vi "GCSArray_regex_select.vi"(0 "GCSArray input string":string, 1 "Selector":T2, 2 "Range":T1, 5 "error in (no error)":errorcluster) -> (14 "Matches":T1[](array[typedef]), 19 "error out":errorcluster)   [LabVIEW 2026]
doc: "Performs the same task as GCSArray_regex_matches.vi, but it returns the found indices as an array of range objects instead of an array of text strings."
uses:
  GCSArray_regex_selector.ctl
  GCSArray_regex_range.ctl
  <vilib>/regexp/Match Regular Expression.xnode
panel:
  # "Select parts ('Selector') of a GCSArray ('Input string')\nand return all found entry ranges ('Matches')."
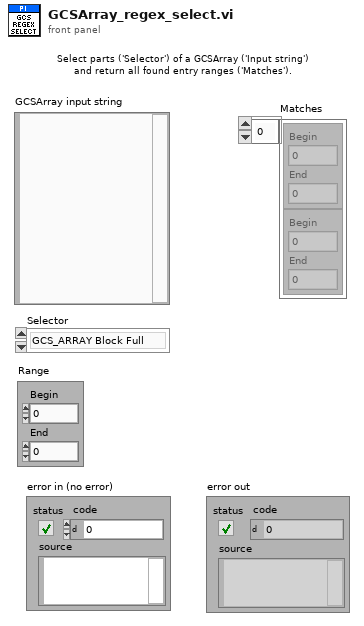
[diagram p1: front panel]
types:
  T1 = typedef "GCSArray_regex_range.ctl" = cluster{"Begin":i32, "End":i32}
  T2 = typedef "GCSArray_regex_selector.ctl" = enum16{"GCS_ARRAY Block Full", "GCS_ARRAY Block ID", "GCS_ARRAY Block Header", "GCS_ARRAY Block Data", "GCS_ARRAY Identifier", "GCS_ARRAY Remark", "GCS_ARRAY Version", "GCS_ARRAY Dimension", "GCS_ARRAY Type", "GCS_ARRAY Separator", "GCS_ARRAY NData", "GCS_ARRAY NData%", "GCS_ARRAY NData% Keyword", "GCS_ARRAY Name%", "GCS_ARRAY Name% Keyword", "GCS_ARRAY Start%", "GCS_ARRAY Start% Keyword", "GCS_ARRAY End%", "GCS_ARRAY End% Keyword", "GCS_ARRAY Delta%", "GCS_ARRAY Delta% Keword", "GCS_ARRAY Sample Time", "GCS_ARRAY Unit of transmitted value%", "GCS_ARRAY Trans_Unit% Keyword", "GCS_ARRAY Trans_Unit% = RAW Keyword", "GCS_ARRAY Unit of displayed value%", "GCS_ARRAY Disp_Unit% Keyword", "GCS_ARRAY Nominator%", "GCS_ARRAY Ratio_Nom% Keyword", "GCS_ARRAY Denominator%", "GCS_ARRAY Ratio_Denom% Keyword", "GCS_ARRAY End of Header", "GCS_ARRAY Empty line of Header"}
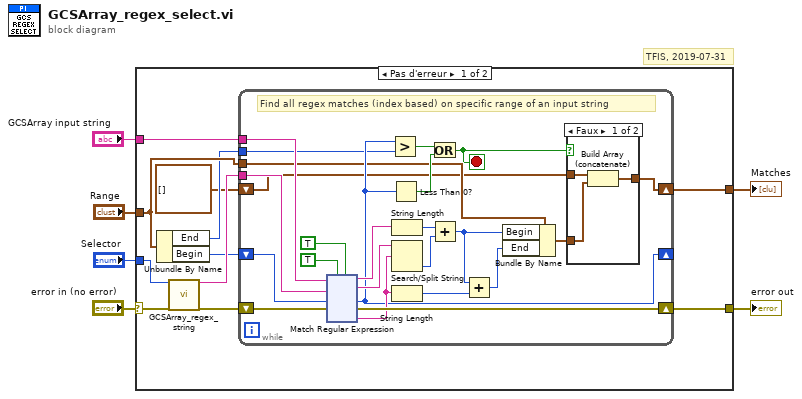
[diagram p0: block diagram]
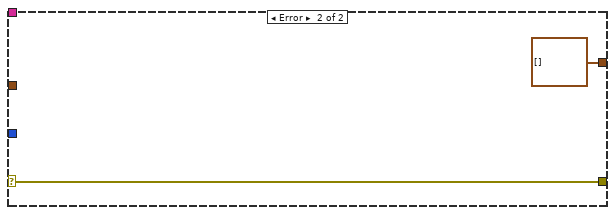
[diagram p3: hidden frame]
diagram:
  # "TFIS, 2019-07-31"
  n1 = case shown="Pas d'erreur" "error in (no error)" {
    selector: "error in (no error)" -> [w13 w166]
    tunnel: [w17 w166] -> w5
    tunnel: "GCSArray input string" -> [w16 _]
    tunnel: "Selector" -> [w15 _]
    tunnel: "Range" -> [w11 _]
    tunnel: [w9 T1[] []] -> w1
    frame No Error {
      n2 = Unbundle By Name(w11) -> ("End"=w8:i32, "Begin"=w10:i32)
      n3 = call "GCSArray_regex_string.vi"("Selector"=w15, "error in (no error)"=w13) -> ("Regex string"=w14:string, "error out"=w12:errorcluster)  [unwired: 16 out]
      n4 = while {
        shift-right: [w39] -> w17
        shift-left: w12 -> [w26]
        shift-right: [w31] -> _
        shift-left: w10 -> [w38]
        tunnel: w16 -> [w28]
        tunnel: w14 -> [w27]
        tunnel: w11 -> [w25]
        tunnel: w8 -> [w21]
        shift-right: [w19] -> w9
        shift-left: T1[] [] ("Array") -> [w20]
        stop <- w18 stop-if-true
        # "Find all regex matches (index based) on specific range of an input string"
        n5 = xnode "Match Regular Expression"("chaîne en entrée"=w28, "expression régulière"=w27, "offset (0)"=w38, "entrée d'erreur"=w26, "ignorer la casse ? (F)"=TRUE ("ignore case? (F)"), "multiligne ? (F)"=TRUE ("multiline? (F)")) -> ("avant la correspondance"=w37:string, "toute l'expression"=w36:string, "offset après correspondance"=w31:i32, "sortie d'erreur"=w39:errorcluster, "correspondance partielle 1"=w33:string)  [unwired: 1 out]
        n6 = Greater?(x=w31, y=w21) -> (0:w30:bool)
        n7 = Less Than 0?(x=w31) -> (x < 0?=w29:bool)
        n8 = String Length(string=w37) -> (length=w35:i32)
        n9 = Search/Split String(string=w36, search string/char (-)=w33) -> (offset of match=w34:i32)  [unwired: 3 out]
        n10 = String Length(string=w33) -> (length=w32:i32)
        n11 = Or(x=w30, y=w29) -> (x .or. y?=w18:bool)
        n12 = Add(x=w35, y=w34) -> (x+y=w23:i32)
        n13 = Add(x=w23, y=w32) -> (x+y=w22:i32)
        n14 = Bundle By Name(cluster=w25, "Begin"=w23, "End"=w22) -> (w24:T1)
        n15 = case shown="Faux" w18 {
          tunnel: w20 -> [w43 w45]
          tunnel: w24 -> [w42 _]
          tunnel: [w44 w45] -> w19
          frame False {
            n16 = Build Array (concatenate)(w43, w42) -> (w44:T1[])
          }
          frame True {
          }
        }
      }
    }
    frame Error {
    }
  }
  "error out" <- w5
  "Matches" <- w1
